vi "Test Read DAT and TDMS.vi"() -> ()   [LabVIEW 2019]
uses:
  src/LV-Data/Typedefs/Dictionary--cluster.ctl
  9b17270d-5d0c-4365-9a1f-7ea8eb203ad9.vi
  06af5cf2-6c13-4970-920c-06c6a4bda324.vi
  1d0c72e7-2fd5-4ada-9d2c-d8c7b4a58351.vi
  <userlib>/_OpenG.lib/file/file.llb/Build Path - File Names Array__ogtk.vi
  <vilib>/Utility/error.llb/Error Cluster From Error Code.vi
  src/LV-Data/LV-Data.lvclass
panel:
  out "XY Graph 3":cluster{dbl[], dbl[]}[](graph)
  out "XY Graph 2":cluster{dbl[], dbl[]}[](graph)
  out "XY Graph":cluster{dbl[], dbl[]}[](graph)
  out "TDMS Folder":cluster{"Data (Dictionary)":T1[]}[](array[cluster])
  out "TDMS File":cluster{"Data (Dictionary)":T1[]}[](array[cluster])
  out "Dat File":cluster{"Data (Dictionary)":T1[]}[](array[cluster])
  out "read tdms folder":dbl=0.017194199841469526
  out "read tdms file":dbl=0.3189365998841822
  out "read dat":dbl=0.32978839986026287
  in  "TDMS Folder":path=path "G:/.shortcut-targets-by-id/0B8-gGFa6hkR4XzJJMDlqZXVKRk0/ansom/Data/MNK/SA40379A.20221206/01 - Vtg test"
  in  "TDMS File":path=path "G:/.shortcut-targets-by-id/0B8-gGFa6hkR4XzJJMDlqZXVKRk0/ansom/Data/PPMSDAQ/2020/PPMS 1/SA40244A.20210723/05-Vbg sweep/SA40244A.20210723.000000.tdms"
  in  "DAT file":path=path "G:/.shortcut-targets-by-id/0B8-gGFa6hkR4XzJJMDlqZXVKRk0/ansom/Data/MNK/SA40286K.20220307/00-Cooldown/SA40286K.20220307.000000.dat"
  # "Array (1) of Cluster of Array of Dictionary [Key, Data Array]"
  # "Array (1) of Cluster of  Array of Dictionary [Key, Dictionary [Key, Data Array]]"
  # "Array (N) of Cluster of Array of Dictionary [Key, Dictionary [Key, Data Array]]"
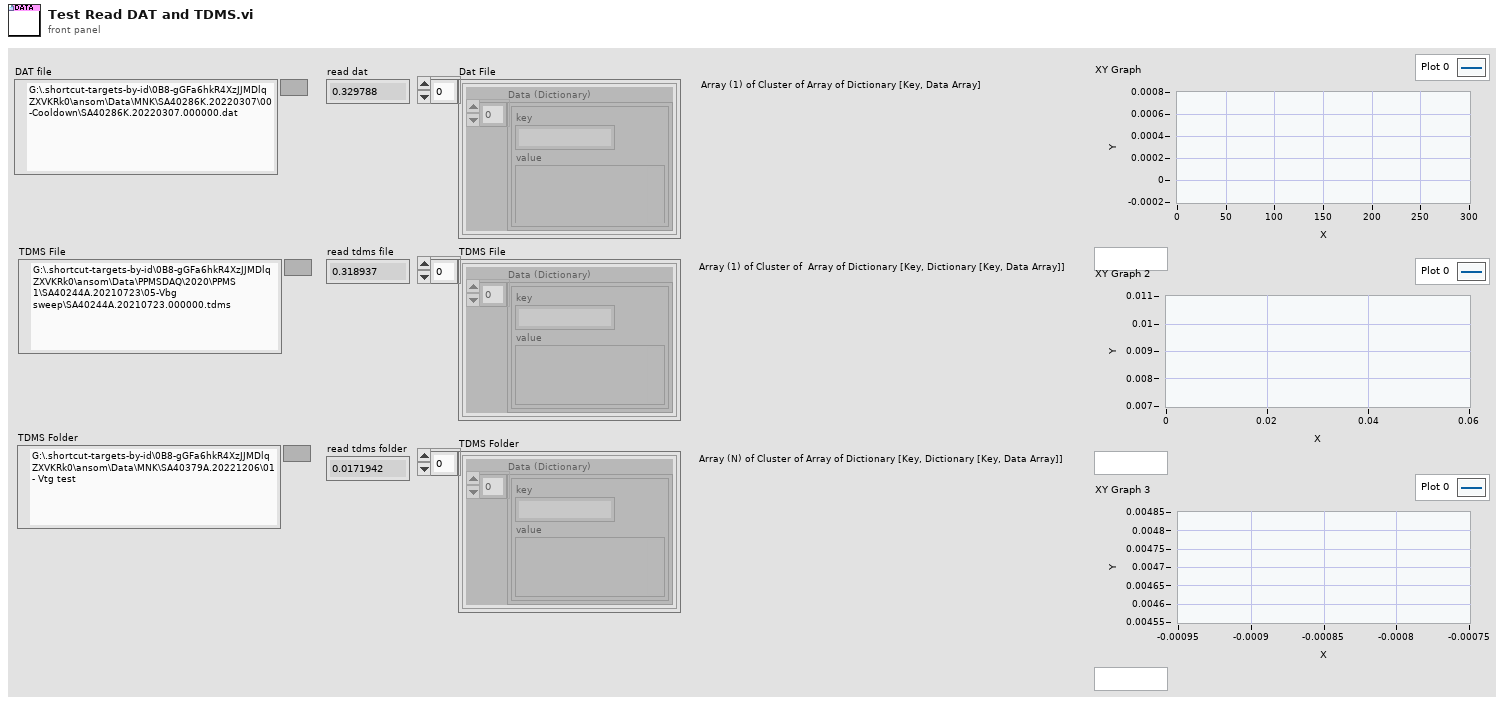
[diagram p1: front panel]
types:
  T1 = typedef "LV-Data.lvclass/Dictionary--cluster.ctl" = cluster{"key":string, "value":variant}
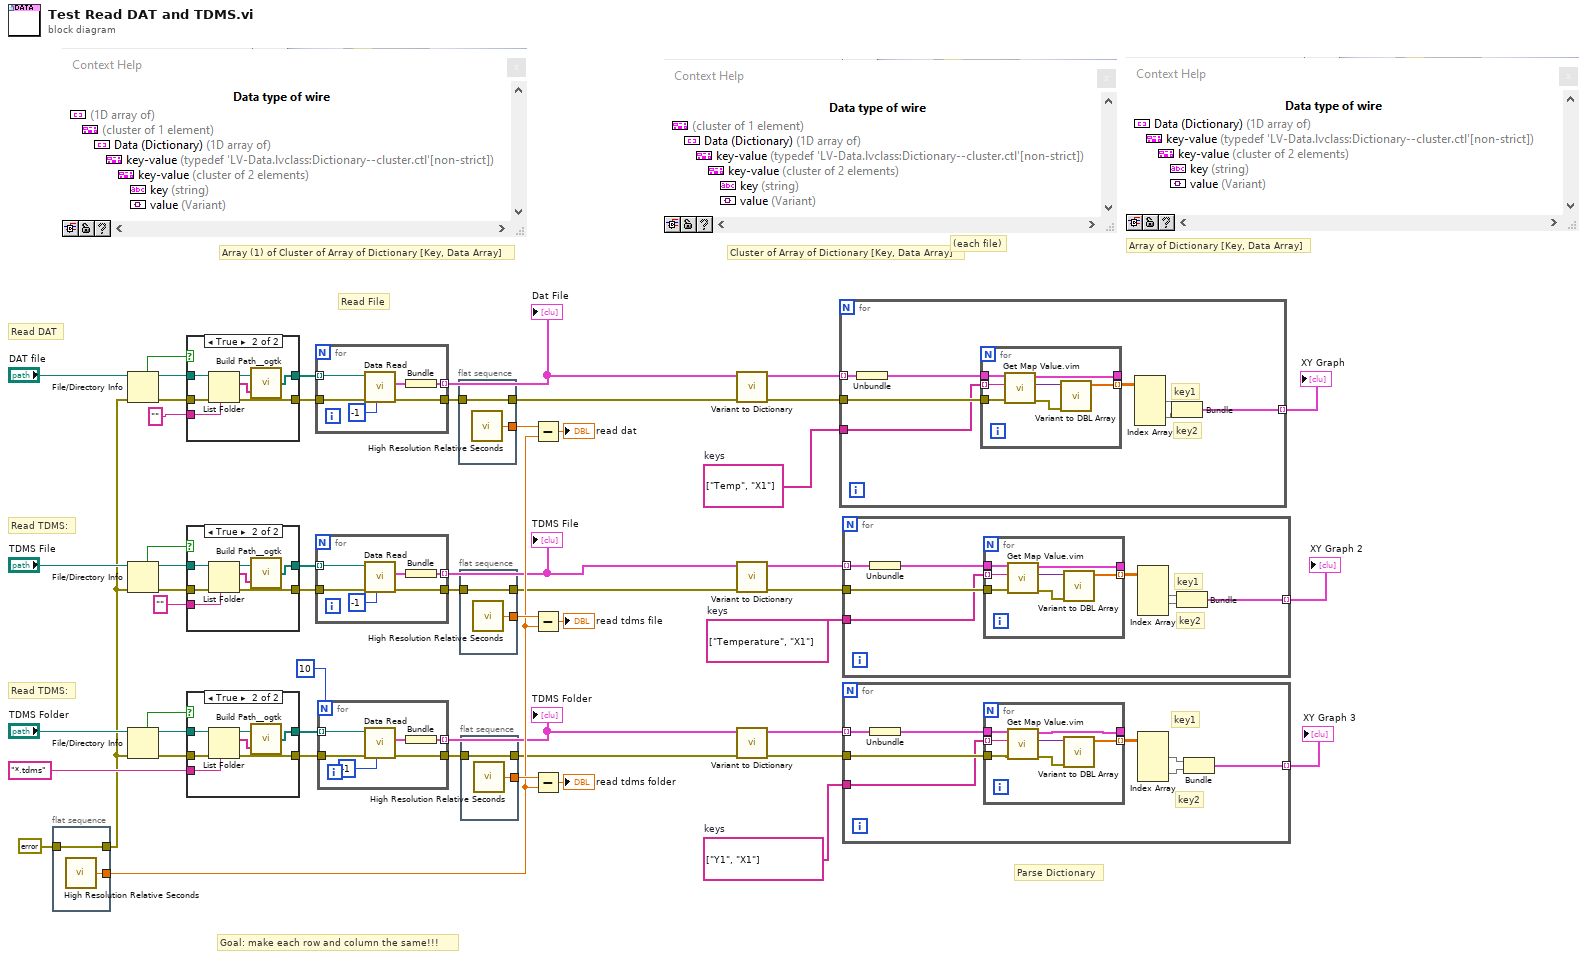
[diagram p0: block diagram]
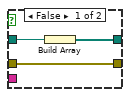
[diagram p2: hidden frame]
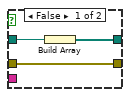
[diagram p3: hidden frame]
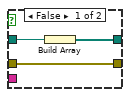
[diagram p4: hidden frame]
diagram:
  w18 = string[] ["Temperature", "X1"]  # keys
  w19 = string[] ["Temp", "X1"]  # keys
  w17 = string[] ["Y1", "X1"]  # keys
  # "(each file)"
  # "Array of Dictionary [Key, Data Array]"
  # "Cluster of Array of Dictionary [Key, Data Array]"
  # "Array (1) of Cluster of Array of Dictionary [Key, Data Array]"
  # "Parse Dictionary"
  # "Goal: make each row and column the same!!!"
  # "Read File"
  # "Read DAT"
  # "Read TDMS:"
  # "Read TDMS:"
  n1 = flat-sequence {
    tunnel: [w54] -> w30
    tunnel: errorcluster {"status"=FALSE, "code"=0, "source"=""} ("error in (no error)") -> [w54]
    tunnel: [w53] -> w23
    frame #0 {
      n2 = call <vilib>:"High Resolution Relative Seconds.vi"() -> ("relative seconds"=w53:dbl)
    }
  }
  n3 = File/Directory Info(path="DAT file", error in=w30) -> (path out=w41:path, directory=w39:bool, error out=w40:errorcluster)  [unwired: 4 out]
  n4 = File/Directory Info(path="TDMS File", error in=w30) -> (path out=w43:path, directory=w45:bool, error out=w44:errorcluster)  [unwired: 4 out]
  n5 = File/Directory Info(path="TDMS Folder", error in=w30) -> (path out=w51:path, directory=w46:bool, error out=w49:errorcluster)  [unwired: 4 out]
  n6 = case shown="True" w39 {
    tunnel: w41 -> [w57 w64]
    tunnel: [w56 w63] -> w36
    tunnel: w40 -> [w55 w62]
    tunnel: [w55 w61] -> w35
    tunnel: "" ("pattern") -> [_ w60]
    frame False {
      n7 = Build Array(w57) -> (w56:path[])
    }
    frame True {
      n8 = List Folder(path=w64, pattern=w60, error in=w62) -> (path out=w59:path, filenames=w58:string[], error out=w61:errorcluster)  [unwired: 1 in, 1 out]
      n9 = call-poly <userlib>:"Build Path__ogtk.vi"("name or relative path"=w58, "base path"=w59) -> ("appended path"=w63:path[])
    }
  }
  n10 = case shown="True" w45 {
    tunnel: w43 -> [w67 w74]
    tunnel: [w66 w73] -> w42
    tunnel: w44 -> [w65 w72]
    tunnel: [w65 w71] -> w34
    tunnel: "" ("pattern") -> [_ w70]
    frame False {
      n11 = Build Array(w67) -> (w66:path[])
    }
    frame True {
      n12 = List Folder(path=w74, pattern=w70, error in=w72) -> (path out=w69:path, filenames=w68:string[], error out=w71:errorcluster)  [unwired: 1 in, 1 out]
      n13 = call-poly <userlib>:"Build Path__ogtk.vi"("name or relative path"=w68, "base path"=w69) -> ("appended path"=w73:path[])
    }
  }
  n14 = case shown="True" w46 {
    tunnel: w51 -> [w77 w84]
    tunnel: [w76 w83] -> w50
    tunnel: w49 -> [w75 w82]
    tunnel: [w75 w81] -> w48
    tunnel: "*.tdms" ("pattern") -> [_ w80]
    frame False {
      n15 = Build Array(w77) -> (w76:path[])
    }
    frame True {
      n16 = List Folder(path=w84, pattern=w80, error in=w82) -> (path out=w79:path, filenames=w78:string[], error out=w81:errorcluster)  [unwired: 1 in, 1 out]
      n17 = call-poly <userlib>:"Build Path__ogtk.vi"("name or relative path"=w78, "base path"=w79) -> ("appended path"=w83:path[])
    }
  }
  n18 = for {
    tunnel: w36 -> [w90] mode=indexing
    tunnel: [w87] -> w10 mode=indexing
    tunnel: [w86] -> w29
    tunnel: w35 -> [w85]
    n19 = call "Data Read.vi"("Append Index"=-1, "error in (no error)"=w85, "path"=w90) -> ("error out"=w86:errorcluster, "Data (Dictionary)"=w88:T1[])  [unwired: 5 in, 2 out]
    n20 = Bundle("Data (Dictionary)"=w88) -> (w87:cluster{"Data (Dictionary)":T1[]})  [unwired: 1 in]
  }
  "Dat File" <- w10
  n21 = for {
    tunnel: w42 -> [w96] mode=indexing
    tunnel: [w93] -> w15 mode=indexing
    tunnel: [w92] -> w28
    tunnel: w34 -> [w91]
    n22 = call "Data Read.vi"("Append Index"=-1, "error in (no error)"=w91, "path"=w96) -> ("error out"=w92:errorcluster, "Data (Dictionary)"=w94:T1[])  [unwired: 5 in, 2 out]
    n23 = Bundle("Data (Dictionary)"=w94) -> (w93:cluster{"Data (Dictionary)":T1[]})  [unwired: 1 in]
  }
  "TDMS File" <- w15
  n24 = for {
    N: 10 -> [_]
    tunnel: w50 -> [w102] mode=indexing
    tunnel: w48 -> [w101]
    tunnel: [w100] -> w6 mode=indexing
    tunnel: [w98] -> w27
    n25 = call "Data Read.vi"("Append Index"=-1, "error in (no error)"=w101, "path"=w102) -> ("error out"=w98:errorcluster, "Data (Dictionary)"=w99:T1[])  [unwired: 5 in, 2 out]
    n26 = Bundle("Data (Dictionary)"=w99) -> (w100:cluster{"Data (Dictionary)":T1[]})  [unwired: 1 in]
  }
  "TDMS Folder" <- w6
  n27 = flat-sequence {
    tunnel: [w104] -> w11
    tunnel: w29 -> [w104]
    tunnel: [w103] -> w26
    frame #0 {
      n28 = call <vilib>:"High Resolution Relative Seconds.vi"() -> ("relative seconds"=w103:dbl)
    }
  }
  n29 = flat-sequence {
    tunnel: [w106] -> w13
    tunnel: w28 -> [w106]
    tunnel: [w105] -> w25
    frame #0 {
      n30 = call <vilib>:"High Resolution Relative Seconds.vi"() -> ("relative seconds"=w105:dbl)
    }
  }
  n31 = flat-sequence {
    tunnel: [w108] -> w7
    tunnel: w27 -> [w108]
    tunnel: [w107] -> w24
    frame #0 {
      n32 = call <vilib>:"High Resolution Relative Seconds.vi"() -> ("relative seconds"=w107:dbl)
    }
  }
  n33 = Subtract(x=w26, y=w23) -> (x-y=→"read dat":dbl)
  n34 = Subtract(x=w25, y=w23) -> (x-y=→"read tdms file":dbl)
  n35 = Subtract(x=w24, y=w23) -> (x-y=→"read tdms folder":dbl)
  n36 = call "Variant to Dictionary.vi"("error in (no error)"=w11, "Array in"=w10) -> ("error out"=w9:errorcluster, "Array out"=w8:cluster{"Data (Dictionary)":T1[]}[])  [unwired: 8 in]
  n37 = call "Variant to Dictionary.vi"("error in (no error)"=w13, "Array in"=w15) -> ("error out"=w14:errorcluster, "Array out"=w12:cluster{"Data (Dictionary)":T1[]}[])  [unwired: 8 in]
  n38 = call "Variant to Dictionary.vi"("error in (no error)"=w7, "Array in"=w6) -> ("error out"=w5:errorcluster, "Array out"=w4:cluster{"Data (Dictionary)":T1[]}[])  [unwired: 8 in]
  n39 = for {
    tunnel: w8 -> [w116] mode=indexing
    tunnel: w9 -> [w114]
    tunnel: w19 -> [w113]
    tunnel: [w109] -> w3 mode=indexing
    # "key2"
    # "key1"
    n40 = Unbundle(w116) -> ("Data (Dictionary)"=w115:T1[])
    n41 = for {
      tunnel: w113 -> [w121] mode=indexing
      tunnel: [w119] -> w112 mode=indexing
      tunnel: w114 -> [w118]
      tunnel: w115 -> [w120]
      tunnel: [w117] -> _
      n42 = call "Get Map Value.vim"("error in (no error)"=w118, "Key"=w121, "map in"=w120) -> ("error out"=w122:errorcluster, "value"=w123:variant, "map out"=w117:T1[])  [unwired: 6 in]
      n43 = call "Variant to DBL Array.vi"("error in (no error)"=w122, "Data (Variant)"=w123) -> ("1D Array"=w119:dbl[])  [unwired: 7 in, 2 out]
    }
    n44 = Index Array(array=w112) -> (element #1=w111:dbl[], element #2=w110:dbl[])  [unwired: 4 in]
    n45 = Bundle("1D Array"=w111, "1D Array"=w110) -> (w109:cluster{"1D Array":dbl[], "1D Array":dbl[]})  [unwired: 1 in]
  }
  "XY Graph" <- w3
  n46 = for {
    tunnel: w12 -> [w131] mode=indexing
    tunnel: w14 -> [w129]
    tunnel: w18 -> [w128]
    tunnel: [w124] -> w2 mode=indexing
    # "key2"
    # "key1"
    n47 = Unbundle(w131) -> ("Data (Dictionary)"=w130:T1[])
    n48 = for {
      tunnel: w128 -> [w136] mode=indexing
      tunnel: [w134] -> w127 mode=indexing
      tunnel: w129 -> [w133]
      tunnel: w130 -> [w135]
      tunnel: [w132] -> _
      n49 = call "Get Map Value.vim"("error in (no error)"=w133, "Key"=w136, "map in"=w135) -> ("error out"=w137:errorcluster, "value"=w138:variant, "map out"=w132:T1[])  [unwired: 6 in]
      n50 = call "Variant to DBL Array.vi"("error in (no error)"=w137, "Data (Variant)"=w138) -> ("1D Array"=w134:dbl[])  [unwired: 7 in, 2 out]
    }
    n51 = Index Array(array=w127) -> (element #1=w126:dbl[], element #2=w125:dbl[])  [unwired: 4 in]
    n52 = Bundle("1D Array"=w126, "1D Array"=w125) -> (w124:cluster{"1D Array":dbl[], "1D Array":dbl[]})  [unwired: 1 in]
  }
  "XY Graph 2" <- w2
  n53 = for {
    tunnel: w17 -> [w143]
    tunnel: w4 -> [w146] mode=indexing
    tunnel: w5 -> [w144]
    tunnel: [w139] -> w1 mode=indexing
    # "key2"
    # "key1"
    n54 = Unbundle(w146) -> ("Data (Dictionary)"=w145:T1[])
    n55 = for {
      tunnel: w143 -> [w151] mode=indexing
      tunnel: [w148] -> w142 mode=indexing
      tunnel: w144 -> [w147]
      tunnel: w145 -> [w150]
      tunnel: [w149] -> _
      n56 = call "Get Map Value.vim"("error in (no error)"=w147, "Key"=w151, "map in"=w150) -> ("error out"=w152:errorcluster, "value"=w153:variant, "map out"=w149:T1[])  [unwired: 6 in]
      n57 = call "Variant to DBL Array.vi"("error in (no error)"=w152, "Data (Variant)"=w153) -> ("1D Array"=w148:dbl[])  [unwired: 7 in, 2 out]
    }
    n58 = Index Array(array=w142) -> (element #1=w140:dbl[], element #2=w141:dbl[])  [unwired: 4 in]
    n59 = Bundle("1D Array"=w140, "1D Array"=w141) -> (w139:cluster{"1D Array":dbl[], "1D Array":dbl[]})  [unwired: 1 in]
  }
  "XY Graph 3" <- w1
